vi "Test.vi"(10 "Bit to test":u8, 11 "Data_In":u16 format="%.0b") -> (2 "bit value":bool, 3 "Data_Out":u16 format="%.0b")   [LabVIEW 2017, in "Bit Manipulation.lvlib"]
uses:
  Bit Manipulation.lvlib
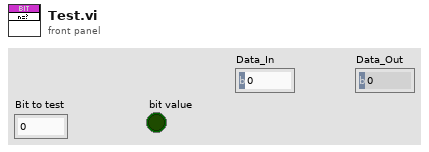
[diagram p1: front panel]
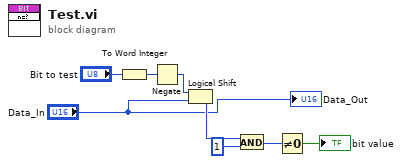
[diagram p0: block diagram]
diagram:
  n1 = To Word Integer(number="Bit to test") -> (16bit integer=w7:i16)
  n2 = Negate(x=w7) -> (-x=w6:i16)
  n3 = Logical Shift(y=w6, x="Data_In") -> (x << y=w5:u16)
  n4 = And(x=w5, y=u16 1) -> (x .and. y?=w3:u16)
  n5 = Not Equal To 0?(x=w3) -> (x != 0?=→"bit value":bool)
  "Data_Out" <- "Data_In"
